vi "获取充放电量信息.vi"(8 "error in (no error)":errorcluster, 11 "MB session in":refnum<class "MB_Master.lvclass">) -> (0 "error out":errorcluster, 2 "充放电信息":T1, 3 "MB session out":refnum<class "MB_Master.lvclass">)   [LabVIEW 2016, in "环境动力监测库.lvlib"]
uses:
  <vilib>/Plasmionique/MB Master/MB_Master/MB_Master.lvclass
  <vilib>/Plasmionique/MB Master/MB Master.lvlib
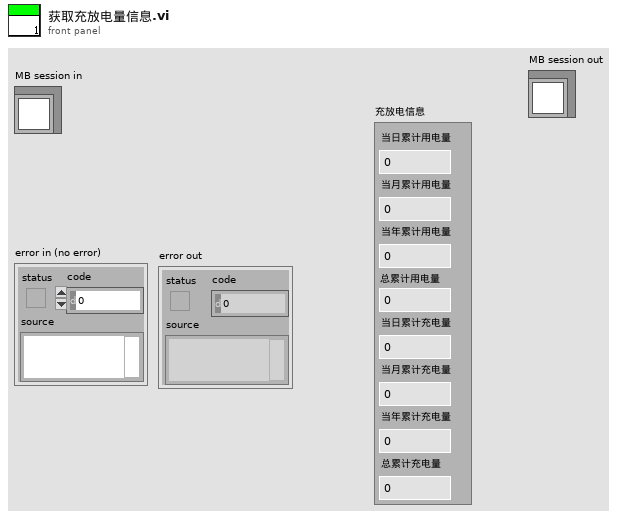
[diagram p1: front panel]
types:
  T1 = cluster{"当日累计用电量":sgl, "当月累计用电量":sgl, "当年累计用电量":sgl, "总累计用电量":sgl, "当日累计充电量":sgl, "当月累计充电量":sgl, "当年累计充电量":sgl, "总累计充电量":sgl}
  T2 = cluster{"[0]":dbl, "[1]":dbl, "[2]":dbl, "[3]":dbl, "[4]":dbl, "[5]":dbl, "[6]":dbl, "[7]":dbl}
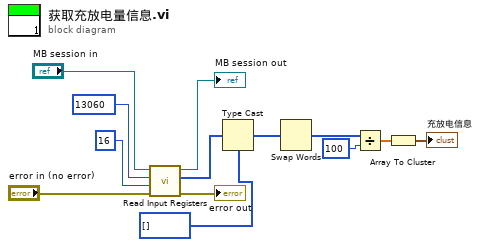
[diagram p0: block diagram]
diagram:
  n1 = call <vilib>:"Read Input Registers.vi"("error in (no error)"="error in (no error)", "quantity"=u16 16, "starting address"=u16 13060, "MB session in"="MB session in") -> ("error out"=→"error out":errorcluster, "Registers"=w6:u16[], "MB session out"=→"MB session out":refnum<class "MB_Master.lvclass">)  [unwired: 5 in]
  n2 = Type Cast(type=i32[] [], x=w6) -> (*(type *) &x=w9:i32[])
  n3 = Swap Words(1:w9) -> (0:w2:i32[])
  n4 = Divide(x=w2, y=100) -> (x/y=w3:dbl[])
  n5 = Array To Cluster(array=w3) -> (cluster=→"充放电信息":T2)
